vi "whatsVisibleTI.vi"(11 "TIplotInfoArray":T1(array[cluster])) -> (1 "Targets Visible":bool[](array[boolean]), 3 "Basics Visible":bool[](array[boolean]))   [LabVIEW 2014]
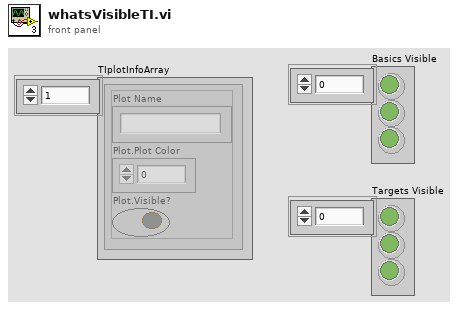
[diagram p1: front panel]
types:
  T1 = cluster{"Plot Name":string, "Plot.Plot Color":u32, "Plot.Visible?":bool}[]
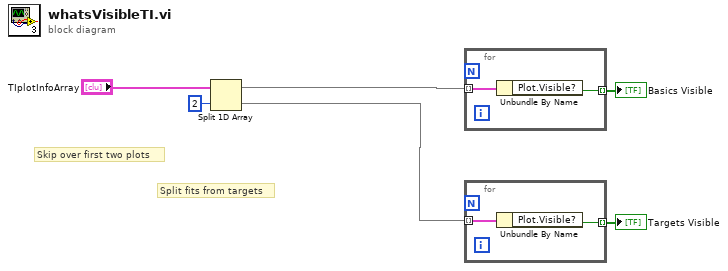
[diagram p0: block diagram]
diagram:
  # "Split fits from targets"
  # "Skip over first two plots"
  n1 = Split 1D Array(array="TIplotInfoArray", index=2) -> (first subarray=w1:T1, second subarray=w3:T1)
  n2 = for {
    tunnel: w1 -> [w8] mode=indexing
    tunnel: [w7] -> w2 mode=indexing
    n3 = Unbundle By Name(w8) -> ("Plot.Visible?"=w7:bool)
  }
  "Basics Visible" <- w2
  n4 = for {
    tunnel: w3 -> [w10] mode=indexing
    tunnel: [w9] -> w4 mode=indexing
    n5 = Unbundle By Name(w10) -> ("Plot.Visible?"=w9:bool)
  }
  "Targets Visible" <- w4
